vi "Named Service TCP Server.vi"() -> ()   [LabVIEW 2014]
doc: "This VI creates a named service on the first available port.\nWhen a client connects to the server, it responds by sending a string to the client and closes the connection. The VI can be stopped using the STOP button.\n\n<b>Note:</b> This VI is built to work with the Named Service TCP Client.vi in TCP.llb."
panel:
  in  "stop":bool
  out "error out":errorcluster
  in  "error in":errorcluster
  # "Instructions:\n1. Open the Named Service TCP Client.vi\n2. Run this VI first.\n3. Run the Named Service TCP Client.vi second.\n4. Observe the output displayed by the Named Service TCP Client.vi.\n\nNote: This VI is built to work with the Named Service \nTCP Client.vi in TCP.llb."
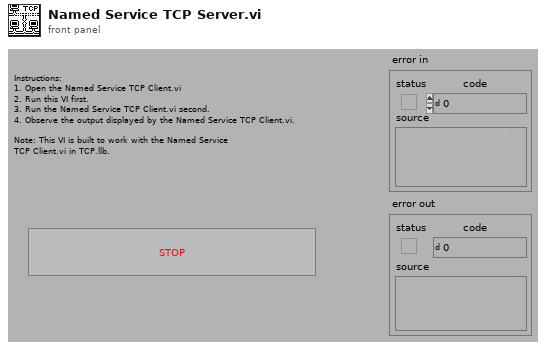
[diagram p1: front panel]
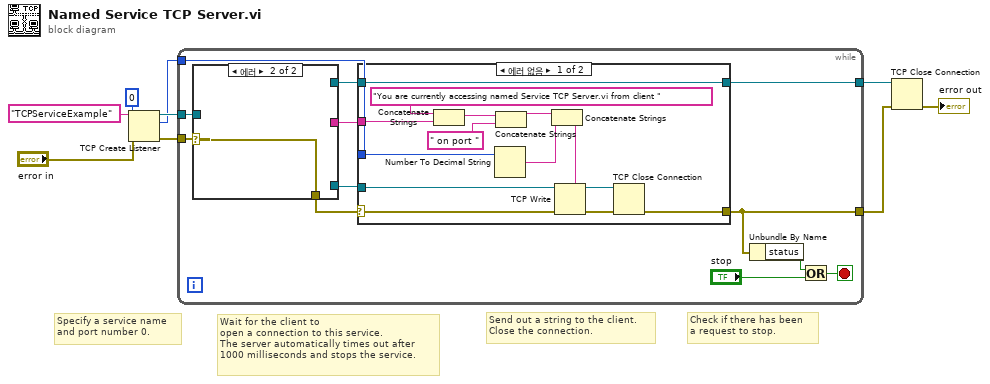
[diagram p0: block diagram]
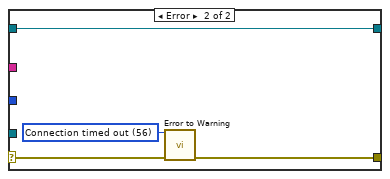
[diagram p2: hidden frame]
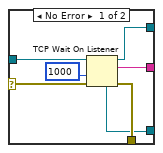
[diagram p3: hidden frame]
diagram:
  # "Check if there has been\na request to stop."
  # "Send out a string to the client.\nClose the connection."
  # "Wait for the client to\nopen a connection to this service.\nThe server automatically times out after \n1000 milliseconds and stops the service."
  # "Specify a service name\nand port number 0."
  n1 = TCP Create Listener(8:"error in", 10:0, 11:"TCPServiceExample") -> (0:w5:errorcluster, 2:w4:u16, 3:w6:refnum<k5>)  [unwired: 2 out]
  n2 = while {
    tunnel: w6 -> [w21]
    tunnel: w5 -> [w18]
    tunnel: [w10] -> w2
    tunnel: w4 -> [w17]
    tunnel: [w15] -> w3
    stop <- w13 stop-if-true
    n3 = case shown="에러" w18 {
      selector: w18 -> [w45 w47]
      tunnel: w21 -> [w46 _]
      tunnel: [w44 w47] -> w14
      tunnel: [w43 _] -> w20
      tunnel: [w42 _] -> w19
      tunnel: [w40 _] -> w16
      frame No Error {
        n4 = TCP Wait On Listener(8:w45, 9:1000, 11:w46) -> (0:w44:errorcluster, 2:w43:string, 3:w40:refnum<k5>, 4:w42:refnum<k5>)  [unwired: 2 out]
      }
      frame Error {
      }
    }
    n5 = case shown="에러 없음" w14 {
      selector: w14 -> [w23 w37]
      tunnel: w20 -> [w34 _]
      tunnel: w17 -> [w31 _]
      tunnel: [w26 w36] -> w10
      tunnel: w19 -> [w27 _]
      tunnel: [w22 w39] -> w15
      tunnel: w16 -> [w22 w39]
      frame No Error {
        n6 = Concatenate Strings("You are currently accessing named Service TCP Server.vi from client " ("String"), w34) -> (w33:string)
        n7 = Number To Decimal String(number=w31) -> (decimal integer string=w30:string)  [unwired: 1 out]
        n8 = Concatenate Strings(w33, " on port " ("String 2")) -> (w29:string)
        n9 = Concatenate Strings(w29, w30) -> (w28:string)
        n10 = TCP Write(connection ID=w27, data in=w28, error in (no error)=w23) -> (connection ID out=w24:refnum<k5>, error out=w25:errorcluster)  [unwired: 2 out]
        n11 = TCP Close Connection(connection ID=w24, error in (no error)=w25) -> (error out=w26:errorcluster)  [unwired: 2 out]
      }
      frame Error {
        w38 = 56 items=["No Error", "Argument Error", "Memory Full", "Out of Zone", "End of File", "File Already Open", "Generic File IO Error", "File Not Found", "File Permission Error", "Disk Full", "Duplicate Path", "Too Many Files Open", "Not Enabled", "Resource File Not Found", "Cannot Add Resource", "Resource Not Found", "Image Not Found", "Image Memory Error", "Pen Does Not Exist", "Config Bad Type", "Config Token Not Found", "Config Parse Error", "Config Memory Error", "Bad External Code Format", "Bad External Code Offset", "External Code Not Present", "Null Window", "Destroy Window Mixup", "Null Menu", "Print Aborted", "Bad Print Record", "Print Driver Error", "Windows Error During Print", "Memory Error During Print", "Print Dialog Error", "Generic Print Error", "Invalid Device Refnum", "Device Not Found", "Device Parameter Error", "Device Unit Error", "Can't Open Device", "Device Call Aborted", "Generic Error", "Cancelled By User", "Object ID Too Low", "Object ID Too High", "Object Not In Heap", "Unknown Heap", "Bad DefProc ID", "DefProc Not In Table", "Message Out Of Range", "Null Method", "Unknown Message", "Manager Call Not Supported", "Bad address", "Connection In progress", "Connection timed out", "Connection is already in progress", "Network attribute not supported", "Network error", "Address in use", "System out of memory", "Connection aborted", "Connection refused", "Connection is not connected", "Connection is already connected", "Connection closed", "Initialize error (interapplication manager)", "Bad occurrence", "Wait on unbound occurrence handler", "Occurrence queue overflow", "Bad path", "Semaphore not signaled", "Unrecognized type (interapplication manager)"] ("1st Error to Convert")
        n12 = call <vilib>:"Error to Warning.vi"("1st Error to Convert"=w38, "error in"=w37) -> ("warning out"=w36:errorcluster)  [unwired: 4 in, 9 out]
      }
    }
    n13 = Unbundle By Name(w10) -> ("status"=w12:bool)
    n14 = Or(x=w12, y="stop") -> (x .or. y?=w13:bool)
  }
  n15 = TCP Close Connection(connection ID=w3, error in (no error)=w2) -> (error out=→"error out":errorcluster)  [unwired: 2 out]
